vi "camera_create_configuration.vi"(3 "error in":errorcluster, 4 "BufferInterval":u32, 5 "Session Out 2":T1) -> (0 "Fehler (Ausgang)":errorcluster, 1 "Session Out":T1, 2 "Ereignisregistrierung (Referenz)":refnum<event-registration>)   [LabVIEW 2009]
uses:
  <vilib>/userDefined/High Color/IMAQdx.ctl
  <vilib>/vision/driver/IMAQdx.llb/IMAQdx Acquisition Mode.ctl
  <vilib>/vision/driver/NI_Vision_Acquisition_Software.lvlib
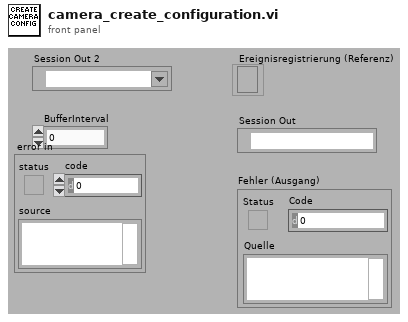
[diagram p1: front panel]
types:
  T1 = typedef "IMAQdx.ctl" = refnum<k21>
  T2 = typedef "NI_Vision_Acquisition_Software.lvlib/IMAQdx Acquisition Mode.ctl" = enum32{"One Shot", "Continuous"}
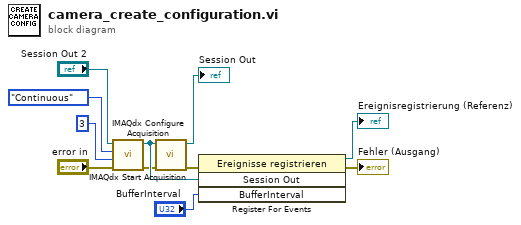
[diagram p0: block diagram]
diagram:
  n1 = call <vilib>:"IMAQdx Configure Acquisition.vi"("error in"="error in", "Number of Buffers"=u32 3, "Continuous?"=IMAQdx_Acquisition_Mode."Continuous", "Session In"="Session Out 2") -> ("error out"=w3:errorcluster, "Session Out"=w5:T1)  [unwired: 6 in]
  n2 = call <vilib>:"IMAQdx Start Acquisition.vi"("error in"=w3, "Session In"=w5) -> ("error out"=w2:errorcluster, "Session Out"=→"Session Out":T1)  [unwired: 8 in]
  n3 = register-events(error in=w2, w5, "BufferInterval") -> (reference out=→"Ereignisregistrierung (Referenz)":refnum<event-registration>, error out=→"Fehler (Ausgang)":errorcluster)  [unwired: 1 in]
